vi "Stop Core.vi"(10 "final error code":i32, 11 "Ex Nested in":refnum<class "SuperActor.lvclass">) -> (3 "Ex Nested out":refnum<class "SuperActor.lvclass">)   [LabVIEW 2015, in "SuperActor.lvclass"]
doc: "(<B>Filename</B>: Actor Framework.lvlib:Actor.lvclass:Stop Core.vi)\n\nDefines what the actor does before it stops. Use the <B>final error code</B> input to determine whether the actor shut down in response to an error.\n\nBy default, this method does nothing. A descendant class may override it to define behavior, such as shutting down any processes the actor initiated in its override of the Actor Core method."
uses:
  SuperActor.lvclass
  Session APIs/CVT/CVT.lvclass
  Session APIs/File Access/Config Data/Config Data.lvclass
  Session APIs/Session Log/System Log.lvclass
  SuperActor.lvclass/SuperActor.ctl
  <vilib>/ActorFramework/Actor/Actor.lvclass
  Session APIs/_Session Fwk/Session - Root.lvclass
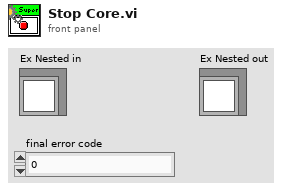
[diagram p1: front panel]
types:
  T1 = typedef "Session - Root.lvclass/Session Handle.ctl" = refnum<data-value>
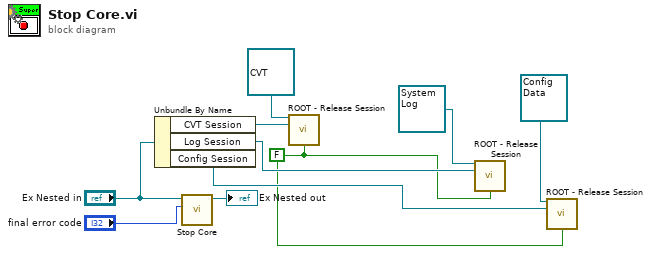
[diagram p0: block diagram]
diagram:
  w1 = FALSE ("force destroy? (F)")
  n1 = Unbundle By Name("Ex Nested in") -> ("CVT Session"=w7:T1, "Log Session"=w5:T1, "Config Session"=w4:T1)
  n2 = call-parent "Stop Core.vi"("final error code"="final error code", "Actor in"="Ex Nested in") -> ("Actor out"=→"Ex Nested out":refnum<class "SuperActor.lvclass">)  [unwired: 9 in]
  n3 = call "ROOT - Release Session.vi"("OBJ - Session in"=refnum<class "CVT.lvclass"> refnum ("CVT"), "Session Handle in"=w7, "force destroy? (F)"=w1) -> ()  [unwired: 11 in, 2 out]
  n4 = call "ROOT - Release Session.vi"("OBJ - Session in"=refnum<class "System Log.lvclass"> refnum ("Sys Log"), "Session Handle in"=w5, "force destroy? (F)"=w1) -> ()  [unwired: 11 in, 2 out]
  n5 = call "ROOT - Release Session.vi"("OBJ - Session in"=refnum<class "Config Data.lvclass"> refnum ("Config Data"), "Session Handle in"=w4, "force destroy? (F)"=w1) -> ()  [unwired: 11 in, 2 out]
